vi "EPR init.vi"(11 "N loops":i32=-1) -> (0 "error out":errorcluster, 1 "ref task out":refnum<k21>, 2 "sig task out":refnum<k21>, 3 "clock task out":refnum<k21>)   [LabVIEW 2012]
uses:
  <vilib>/DAQmx/create/channels.llb/DAQmx Create Channel (CI-Count Edges).vi
  <vilib>/DAQmx/configure/timing.llb/DAQmx Timing (Sample Clock).vi
  <vilib>/DAQmx/create/channels.llb/DAQmx Create Channel (CO-Pulse Generation-Ticks).vi
  <vilib>/DAQmx/configure/timing.llb/DAQmx Timing (Implicit).vi
  <resource>/objmgr/daqmx.rc
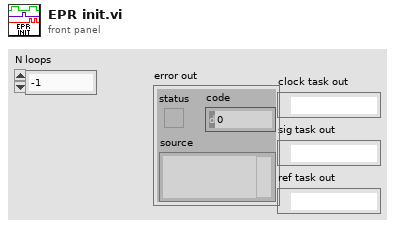
[diagram p1: front panel]
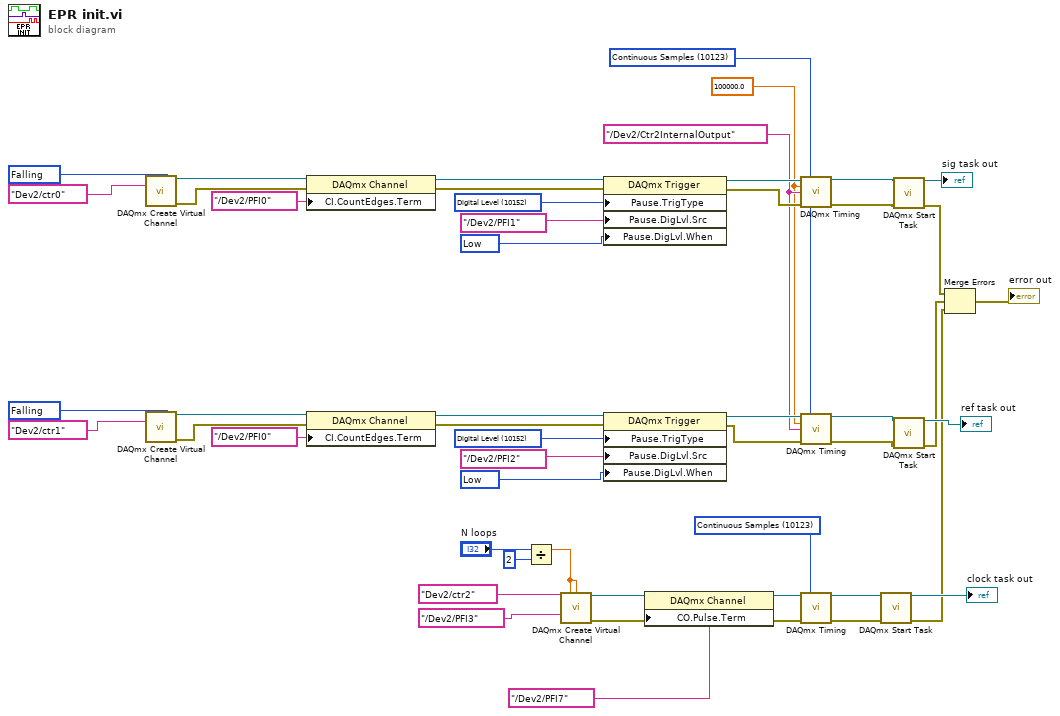
[diagram p0: block diagram]
diagram:
  w7 = 10123 items=["Finite Samples"=10178, "Continuous Samples"=10123, "Hardware Timed Single Point"=12522] ("sample mode")
  w36 = 10214 items=["High"=10192, "Low"=10214] ("Pause.DigLvl.When")
  w38 = 10152 items=["Analog Level"=10101, "Analog Window"=10103, "Digital Level"=10152, "Digital Pattern"=10398, "None"=10230] ("Pause.TrigType")
  w39 = 10171 items=["Rising"=10280, "Falling"=10171] ("edge")
  w26 = tag "/Dev2/Ctr2InternalOutput" ("source")
  w3 = 10123 items=["Finite Samples"=10178, "Continuous Samples"=10123, "Hardware Timed Single Point"=12522] ("sample mode")
  w46 = 10214 items=["High"=10192, "Low"=10214] ("Pause.DigLvl.When")
  w48 = 10152 items=["Analog Level"=10101, "Analog Window"=10103, "Digital Level"=10152, "Digital Pattern"=10398, "None"=10230] ("Pause.TrigType")
  w49 = 10171 items=["Rising"=10280, "Falling"=10171] ("edge")
  w4 = 100000.0 ("rate")
  n1 = call-poly <vilib>:"DAQmx Create Virtual Channel.vi"("edge"=w39, "counter"=tag "Dev2/ctr0") -> ("task out"=w34:refnum<k21>, "error out"=w31:errorcluster)  [unwired: 7 in, 5 out]
  n2 = call-poly <vilib>:"DAQmx Create Virtual Channel.vi"("edge"=w49, "counter"=tag "Dev2/ctr1") -> ("task out"=w44:refnum<k21>, "error out"=w41:errorcluster)  [unwired: 7 in, 5 out]
  n3 = property class="DAQmx Channel"(reference=w34, error in=w31, "CI.CountEdges.Term"=tag "/Dev2/PFI0") -> (reference out=w35:refnum<k21>, error out=w33:errorcluster)
  n4 = property class="DAQmx Channel"(reference=w44, error in=w41, "CI.CountEdges.Term"=tag "/Dev2/PFI0") -> (reference out=w45:refnum<k21>, error out=w43:errorcluster)
  n5 = Divide(x="N loops", y=2) -> (x/y=w13:dbl)
  n6 = call-poly <vilib>:"DAQmx Create Virtual Channel.vi"("high ticks"=w13, "low ticks"=w13, "counter"=tag "Dev2/ctr2", "source of ticks"=tag "/Dev2/PFI3" ("source")) -> ("task out"=w11:refnum<k21>, "error out"=w9:errorcluster)  [unwired: 10 in]
  n7 = property class="DAQmx Trigger"(reference=w35, error in=w33, "Pause.TrigType"=w38, "Pause.DigLvl.Src"=tag "/Dev2/PFI1", "Pause.DigLvl.When"=w36) -> (reference out=w30:refnum<k21>, error out=w29:errorcluster)
  n8 = property class="DAQmx Trigger"(reference=w45, error in=w43, "Pause.TrigType"=w48, "Pause.DigLvl.Src"=tag "/Dev2/PFI2", "Pause.DigLvl.When"=w46) -> (reference out=w28:refnum<k21>, error out=w27:errorcluster)
  n9 = property class="DAQmx Channel"(reference=w11, "CO.Pulse.Term"=tag "/Dev2/PFI7") -> (reference out=w2:refnum<k21>)  [unwired: 1 in, 1 out]
  n10 = call-poly <vilib>:"DAQmx Timing.vi"("task/channels in"=w30, "sample mode"=w3, "rate"=w4, "source"=w26, "error in"=w29) -> ("task out"=w25:refnum<k21>, "error out"=w24:errorcluster)  [unwired: 9 in]
  n11 = call-poly <vilib>:"DAQmx Timing.vi"("task/channels in"=w28, "sample mode"=w3, "rate"=w4, "source"=w26, "error in"=w27) -> ("task out"=w23:refnum<k21>, "error out"=w22:errorcluster)  [unwired: 9 in]
  n12 = call-poly <vilib>:"DAQmx Timing.vi"("task/channels in"=w2, "sample mode"=w7, "error in"=w9) -> ("task out"=w10:refnum<k21>, "error out"=w8:errorcluster)  [unwired: 11 in]
  n13 = call <vilib>:"DAQmx Start Task.vi"("task/channels in"=w10, "error in"=w8) -> ("task out"=→"clock task out":refnum<k21>, "error out"=w5:errorcluster)  [unwired: 12 in]
  n14 = call <vilib>:"DAQmx Start Task.vi"("task/channels in"=w25, "error in"=w24) -> ("task out"=→"sig task out":refnum<k21>, "error out"=w19:errorcluster)  [unwired: 12 out]
  n15 = call <vilib>:"DAQmx Start Task.vi"("task/channels in"=w23, "error in"=w22) -> ("task out"=→"ref task out":refnum<k21>, "error out"=w18:errorcluster)  [unwired: 12 out]
  n16 = Merge Errors(w19, w18, w5) -> (→"error out":errorcluster)
